vi "ModePose.vi"() -> (0 "Pose Mode":T1(ring))   [LabVIEW 2020]
doc: "Manges the pose mode, switching between normal, autonomous sequencer control, initialization, IMU reset only, and manual robot pose pushing from the Dashboard."
uses:
  f3b7fb6a-8615-463b-b779-049d785c3eeb.vi
  GlobalPoseAndTargeting.vi
  GlobalDriverStationData.vi
  GlobalDrivebase.vi
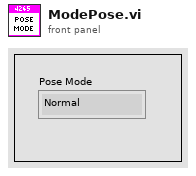
[diagram p1: front panel]
types:
  T1 = enum16{"Normal", "Auto Set", "Reset IMU", "Manual Push", "Init"}
  T2 = enum16{"Center", "North", "NorthWest", "West", "SouthWest", "South", "SouthEast", "East", "NorthEast"}
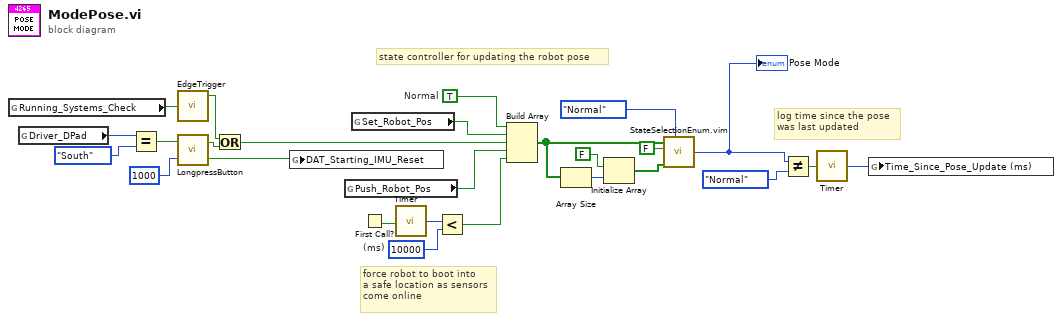
[diagram p0: block diagram]
diagram:
  w9 = u32 10000  # (ms)
  w3 = TRUE  # Normal
  # "force robot to boot into\na safe location as sensors\ncome online"
  # "log time since the pose\nwas last updated"
  # "state controller for updating the robot pose"
  n1 = global read "GlobalDriverStationData.vi" "Running_Systems_Check"() -> (w22:bool)
  n2 = global read "GlobalDriverStationData.vi" "Driver_DPad"() -> (w11:T2)
  n3 = Equal?(x=w11, y=T2."South") -> (x = y?=w12:bool)
  n4 = call "EdgeTrigger.vi"("Input Signal"=w22) -> ("Rising Edge Trigger"=w24:bool)  [unwired: 2 out]
  n5 = call "LongpressButton.vi"("Threshold (ms)"=u32 1000, "Button"=w12) -> ("Starting Press"=w26:bool, "Longpress Button"=w23:bool)
  n6 = Or(x=w24, y=w23) -> (x .or. y?=w25:bool)
  n7 = global write "GlobalDrivebase.vi" "DAT_Starting_IMU_Reset"(w26) -> ()
  n8 = global read "GlobalPoseAndTargeting.vi" "Push_Robot_Pos"() -> (w2:bool)
  n9 = global read "GlobalPoseAndTargeting.vi" "Set_Robot_Pos"() -> (w10:bool)
  n10 = First Call?() -> (First Call?: T/F=w6:bool)
  n11 = call "Timer.vi"("Reset Timer"=w6) -> ("Time (ms)"=w7:u32)
  n12 = Less?(x=w7, y=w9) -> (x < y?=w8:bool)
  n13 = Build Array(w3, w10, w25, w2, w8) -> (w17:bool[])
  n14 = Array Size(array=w17) -> (size(s)=w14:i32)
  n15 = Initialize Array(FALSE, w14) -> (w18:bool[])
  n16 = call "StateSelectionEnum.vim"("Enum Def"=T1."Normal", "Disallowed States"=w18, "Enable Edge Trigger"=FALSE, "State Triggers"=w17) -> ("Selected State"=w21:T1)  [unwired: 1 in, 1 out]
  "Pose Mode" <- w21
  n17 = Not Equal?(x=w21, y=T1."Normal") -> (x != y?=w4:bool)
  n18 = call "Timer.vi"("Reset Timer"=w4) -> ("Time (ms)"=w5:u32)
  n19 = global write "GlobalPoseAndTargeting.vi" "Time_Since_Pose_Update (ms)"(w5) -> ()
